vi "Write Connection.vi"(8 "error in (no error)":errorcluster, 10 "Connection Config":T1, 11 "MQTT Client in":refnum<class "MQTT Client.lvclass">) -> (0 "error out":errorcluster, 3 "MQTT Client out":refnum<class "MQTT Client.lvclass">)   [LabVIEW 2020]
uses:
  MQTT Client.lvclass
  mqttTypedef/ConnectionConfig.ctl
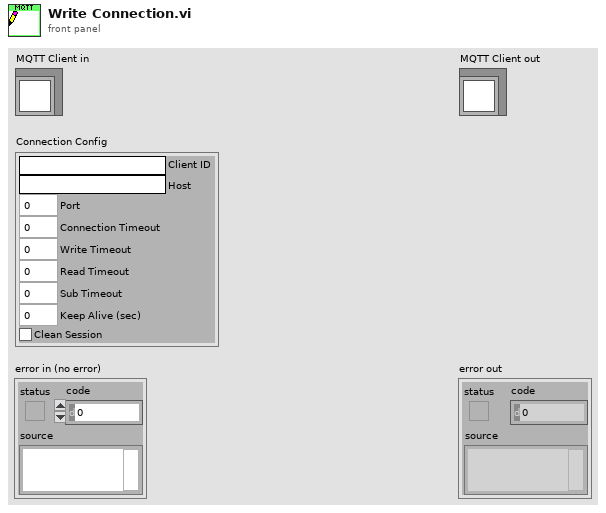
[diagram p1: front panel]
types:
  T1 = typedef "MQTT Client.lvclass/ConnectionConfig.ctl" = cluster{"Client ID":string, "Host":string, "Port":u16, "Connection Timeout":i32, "Write Timeout":i32, "Read Timeout":i32, "Sub Timeout":i32, "Keep Alive (sec)":u16, "Clean Session":bool}
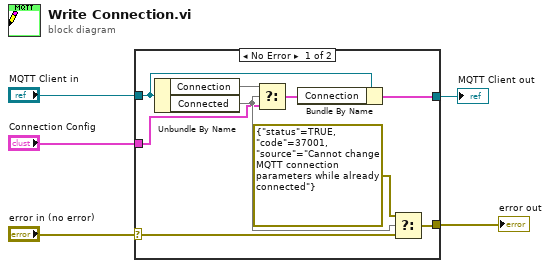
[diagram p0: block diagram]
diagram:
  n1 = case shown="No Error" "error in (no error)" {
    selector: "error in (no error)" -> [w12 w15]
    tunnel: [w11 w15] -> w4
    tunnel: [w14 w16] -> w2
    tunnel: "MQTT Client in" -> [w13 w16]
    tunnel: "Connection Config" -> [w7 _]
    frame No Error {
      n2 = Unbundle By Name(w13) -> ("Connection"=w9, "Connected"=w8)
      n3 = Select(t=w9, s=w8, f=w7) -> (s? t:f=w6:T1)
      n4 = Bundle By Name(cluster=w13, "Connection"=w6) -> (w14:cluster{})
      n5 = Select(t=errorcluster {"status"=TRUE, "code"=37001, "source"="Cannot change MQTT connection parameters while already connected"}, s=w8, f=w12) -> (s? t:f=w11:errorcluster)
    }
    frame Error {
    }
  }
  "error out" <- w4
  "MQTT Client out" <- w2
